vi "PI_GCS2_Simple_Test.vi"() -> ()   [LabVIEW 2026]
doc: "This simple test VI is a stand-alone sample application. Use the \nHelp->Show Context Help menu sequence in the LabVIEW environment to display the Context Help window with the VI and control/indicator descriptions.\n\nSpecify \n- System number (= 1 in a one-system configuration),\n- Interface settings \n- For Interface = RS232: Choose the port number the device is connected to and an appropriate baud rate. \n- For Interface = USB: Choose the appropriate serial number of the device to connect to or if you want to search for the controller.\n- For Interface = TCP/IP: Host address/name and portnumber (default is 50000) of the device to connect to or if you want to search for the controller.\n- Timeout value (in milliseconds)\n\nThen start the VI. The VI will open a connection to the chosen device and query the device for its identification string. The diagram shows how to combine the driver and support VIs for these tasks."
uses:
  Low Level/Communication/Interface Settings.ctl
panel:
  in  "Interface settings":T1={"Interface"=4, "Timeout"=5000, "RS232 settings"={"Portnumber"=1, "Baudrate"=5}, "TCP/IP settings"={"Host address/name"="localhost", "Port"=50000, "Board"=0, "TCP/IP Search?"=TRUE}, "USB settings"={"S/N"="", "USB Search?"=TRUE}, "DaisyChain settings"={"Register DC"=FALSE, "DaisyChain Search?"=TRUE, "Device ID"=1}, "DLL for Device"=0} {"DLL for Device" items=["None", "C-843", "C-844", "E-710", "C-843.PM", "C-865", "E-761", "Mercury", "E-755", "E-753", "C-866", "E-712", "E-725", "E-861", "C-867", "E-517", "E-816", "E-709", "PI_GCS2_DLL", "HydraPollux"]; "Interface" items=["RS232", "RS232 DaisyChain", "USB", "USB DaisyChain", "TCP/IP", "TCP/IP DaisyChain", "DLL"]; "RS232 settings"."Baudrate" items=["9600", "14400", "19200", "38400", "57600", "115200", "230400", "460800"]}
  in  "error in":errorcluster
  in  "System no.":i32=1 min=1 step=1
  out "error out":errorcluster
  out "Identification":string
  # "Simple PI GCS2 Communication Test Program"
  # "Select the interface settings first, then start the VI. The VI will open a connection to the chosen Pi GCS2 device and query \nfor its identification string (*IDN?). See VI and control/indicator information for details."
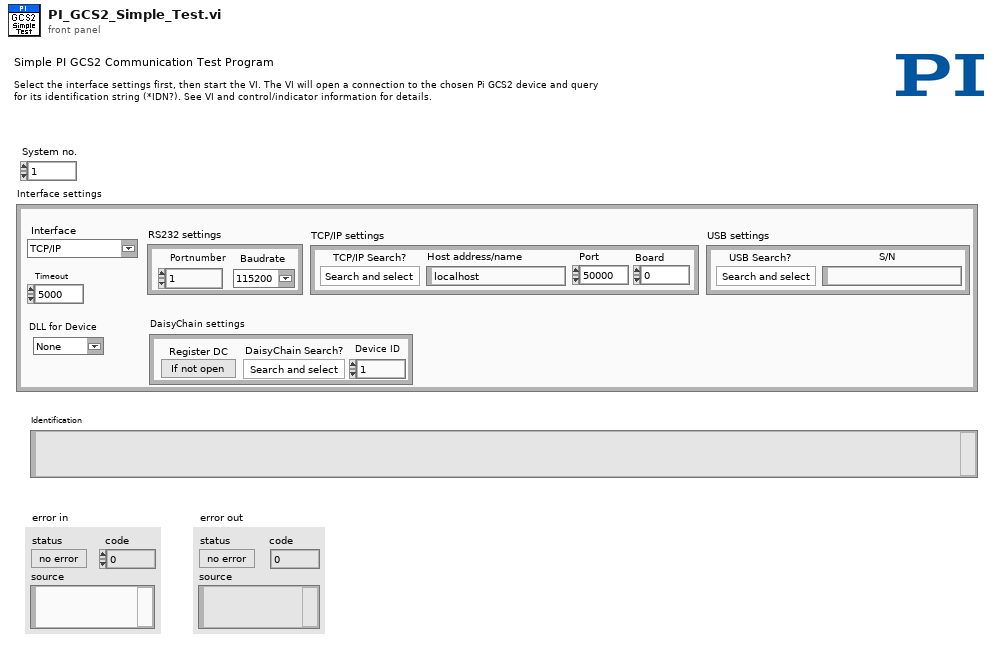
[diagram p1: front panel]
types:
  T1 = typedef "Interface Settings.ctl" = cluster{"Interface":u16, "Timeout":u32, "RS232 settings":cluster{"Portnumber":u8, "Baudrate":u16}, "TCP/IP settings":cluster{"Host address/name":string, "Port":i32, "Board":i32, "TCP/IP Search?":bool}, "USB settings":cluster{"S/N":string, "USB Search?":bool}, "DaisyChain settings":cluster{"Register DC":bool, "DaisyChain Search?":bool, "Device ID":i32}, "DLL for Device":u16}
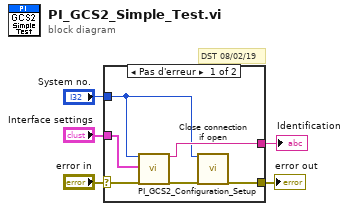
[diagram p0: block diagram]
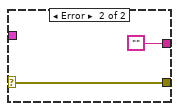
[diagram p2: hidden frame]
diagram:
  # "DST 08/02/19"
  n1 = case shown="Pas d'erreur" "error in" {
    selector: "error in" -> [w10 w13]
    tunnel: [w8 ""] -> w5
    tunnel: [w11 w13] -> w4
    tunnel: "Interface settings" -> [w7 _]
    tunnel: "System no." -> [w6 _]
    frame No Error {
      n2 = call "PI_GCS2_Configuration_Setup.vi"("System no."=w6, "Interface settings"=w7, "error in"=w10) -> ("Identification"=w8:string, "error out"=w9:errorcluster)  [unwired: 5 in, 10 out]
      n3 = call "Close connection if open.vi"("System no."=w6, "error in"=w9) -> ("error out"=w11:errorcluster)  [unwired: 1 in, 16 out]
    }
    frame Error {
    }
  }
  "Identification" <- w5
  "error out" <- w4
